vi "CallTypedefinLib.vi"() -> ()   [LabVIEW 2020]
uses:
  TypeDefInLIb.ctl
  Lib.lvlib
panel:
  in  "Cluster":T1
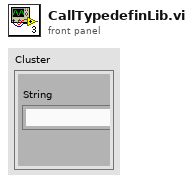
[diagram p1: front panel]
types:
  T1 = typedef "Lib.lvlib/TypeDefInLIb.ctl" = cluster{"String":string}
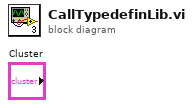
[diagram p0: block diagram]
diagram:
